vi "23384_Davis_Poku_Amankwa_Amankwa.DavisPoku.MNE1201.1.2_348251_1922194810.vi"() -> ()   [LabVIEW 2018]
panel:
  out "Temperture-Tc":dbl
  in  "Temperature-Tf":dbl
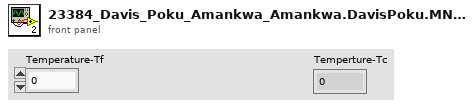
[diagram p1: front panel]
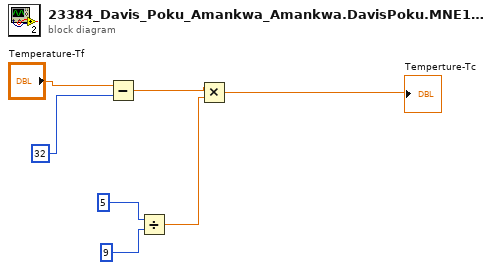
[diagram p0: block diagram]
diagram:
  n1 = Subtract(x="Temperature-Tf", y=32) -> (x-y=w3:dbl)
  n2 = Divide(x=5, y=9) -> (x/y=w2:dbl)
  n3 = Multiply(x=w3, y=w2) -> (x*y=→"Temperture-Tc":dbl)
